vi "Module API.vi"(8 "error in (no error)":errorcluster, 11 "TestModule in":refnum<class "TestModule.lvclass">) -> (0 "error out":errorcluster, 2 "API":refnum<class "API.lvclass">, 3 "TestModule out":refnum<class "TestModule.lvclass">)   [LabVIEW 2020]
uses:
  TestModule.lvclass/TestModule.ctl
  Volatus/API/API.lvclass
  TestModule.lvclass
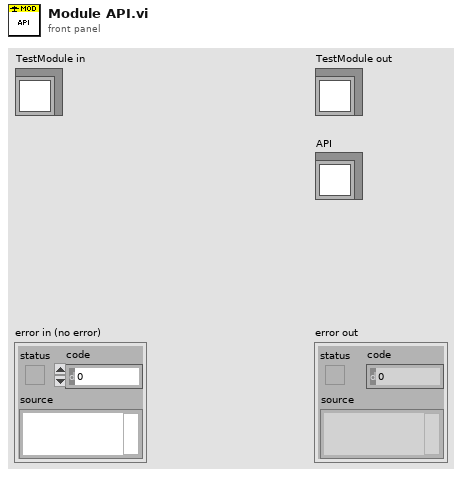
[diagram p1: front panel]
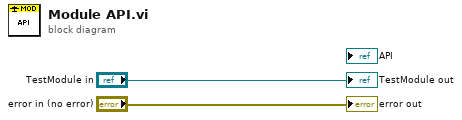
[diagram p0: block diagram]
diagram:
  "error out" <- "error in (no error)"
  "TestModule out" <- "TestModule in"
